vi "Close COM Port.vi"(8 "error in (no error)":errorcluster, 11 "VISA Refnum in":refnum<visa-resource-name>) -> (0 "error out":errorcluster)   [LabVIEW 2017]
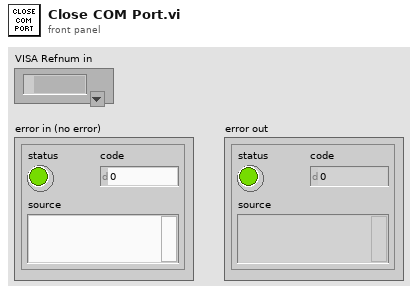
[diagram p1: front panel]
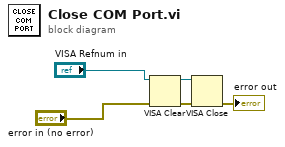
[diagram p0: block diagram]
diagram:
  n1 = VISA Clear(VISA resource name="VISA Refnum in", error in (no error)="error in (no error)") -> (VISA resource name out=w2:refnum<visa-resource-name>, error out=w3:errorcluster)
  n2 = VISA Close(VISA resource name=w2, error in (no error)=w3) -> (error out=→"error out":errorcluster)
